vi "Create.vi"(8 "Error In":errorcluster, 11 "Data":refnum<class "Abstract.lvclass">) -> (0 "Error Out":errorcluster, 3 "Context":refnum<class "Context.lvclass">)   [LabVIEW 2018, in "Toolkit.lvlib" / "Data.lvlib" / "Context.lvclass"]
uses:
  Context.lvclass
  Abstract/Abstract.lvclass
  Context.lvclass/Context.ctl
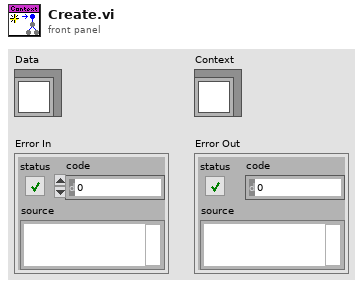
[diagram p1: front panel]
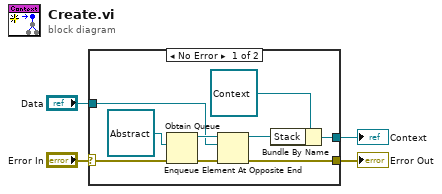
[diagram p0: block diagram]
diagram:
  n1 = case shown="No Error" "Error In" {
    selector: "Error In" -> [w5 w14]
    tunnel: [w10 _] -> w4
    tunnel: [w7 w14] -> w3
    tunnel: "Data" -> [w6 _]
    frame No Error {
      n2 = Obtain Queue(element data type=refnum<class "Abstract.lvclass"> refnum ("Toolkit.lvlib:Data.lvlib:Abstract.lvclass"), error in (no error)=w5) -> (queue out=w11:refnum<queue>, error out=w8:errorcluster)  [unwired: 3 in, 1 out]
      n3 = Enqueue Element At Opposite End(queue=w11, element=w6, error in (no error)=w8) -> (queue out=w9:refnum<queue>, error out=w7:errorcluster)  [unwired: 1 in, 1 out]
      n4 = Bundle By Name(cluster=refnum<class "Context.lvclass"> refnum ("Toolkit.lvlib:Data.lvlib:Context.lvclass"), "Stack"=w9) -> (w10:refnum<class "Context.lvclass">)
    }
    frame Error {
    }
  }
  "Error Out" <- w3
  "Context" <- w4
